vi "Write Digital Port.vi"(8 "error in":errorcluster, 10 "Data":bool[](array[boolean]), 11 "Line(s)":tag="Dev1/port0/line0:7") -> (0 "error out":errorcluster)   [LabVIEW 2015]
doc: "This VI write digital line port.\n\nFor multiple lines use comma to separate channel\nFor Example: Dev1/port0/line0:2,Dev1/port0/line7 // will write DO to line 0 thru 2 and 7\n Set bit 0,1,2,7 to high"
uses:
  <vilib>/DAQmx/write.llb/DAQmx Write (Digital 1D Bool 1Chan 1Samp).vi
  <vilib>/DAQmx/create/channels.llb/DAQmx Create Channel (DO-Digital Output).vi
  <vilib>/DAQmx/miscellaneous.llb/DAQmx Fill In Error Info.vi
panel:
  # "LSB"
  # "MSB"
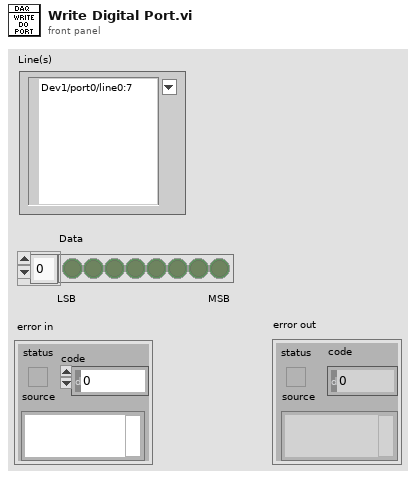
[diagram p1: front panel]
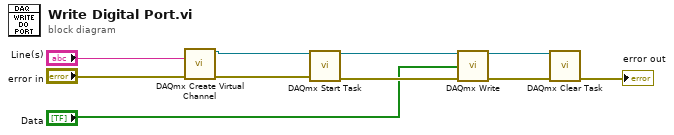
[diagram p0: block diagram]
diagram:
  n1 = call-poly <vilib>:"DAQmx Create Virtual Channel.vi"("lines"="Line(s)", "error in"="error in") -> ("task out"=w5:refnum<k21>, "error out"=w4:errorcluster)  [unwired: 12 in]
  n2 = call <vilib>:"DAQmx Start Task.vi"("task/channels in"=w5, "error in"=w4) -> ("task out"=w7:refnum<k21>, "error out"=w8:errorcluster)  [unwired: 12 in]
  n3 = call-poly <vilib>:"DAQmx Write.vi"("task/channels in"=w7, "data"="Data", "error in"=w8) -> ("task out"=w9:refnum<k21>, "error out"=w10:errorcluster)  [unwired: 10 in, 1 out]
  n4 = call <vilib>:"DAQmx Clear Task.vi"("task in"=w9, "error in"=w10) -> ("error out"=→"error out":errorcluster)  [unwired: 13 in]
